vi "Save-modulation-data.vi"(8 "error in (no error)":errorcluster, 9 "Modulation data":i32[][](array[numeric]), 10 "File path":path) -> (0 "error out":errorcluster)   [LabVIEW 2013, in "MaterialCharacterization.lvlib" / "MC-SM1000.lvclass"]
uses:
  MC-SM1000.lvclass
  <vilib>/Utility/file.llb/Write To Spreadsheet File (I64).vi
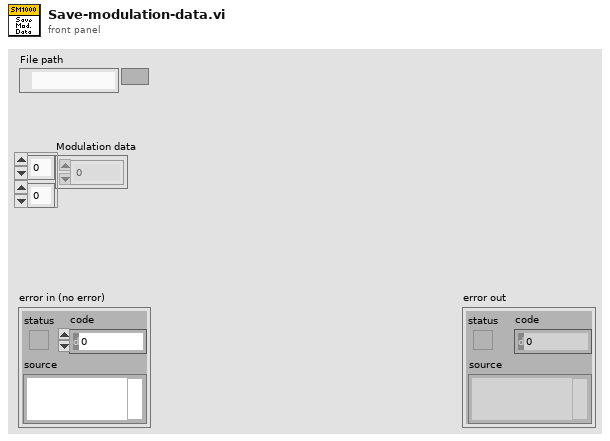
[diagram p1: front panel]
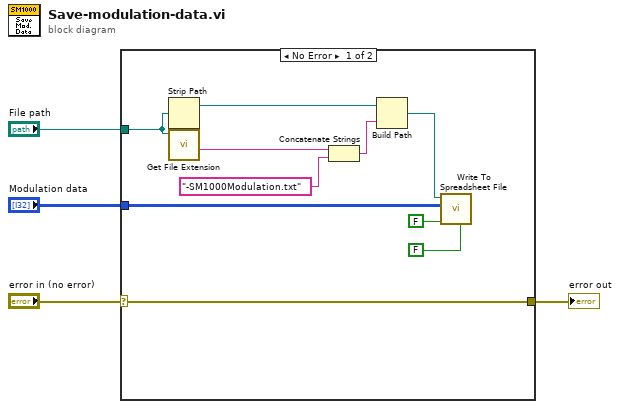
[diagram p0: block diagram]
diagram:
  n1 = case shown="No Error" "error in (no error)" {
    selector: "error in (no error)" -> [w8 w15]
    tunnel: [w8 w15] -> w3
    tunnel: "File path" -> [w7 _]
    tunnel: "Modulation data" -> [w14 _]
    frame No Error {
      n2 = Strip Path(path=w7) -> (stripped path=w12:path)  [unwired: 1 out]
      n3 = call <vilib>:"Get File Extension.vi"("file"=w7) -> ("filename without extension"=w5:string)  [unwired: 7 in, 3 out]
      n4 = Concatenate Strings(w5, "-SM1000Modulation.txt" ("string")) -> (w11:string)
      n5 = Build Path(base path=w12, name or relative path=w11) -> (appended path=w10:path)
      n6 = call-poly <vilib>:"Write To Spreadsheet File.vi"("transpose? (no:F)"=FALSE, "append to file? (new file:F)"=FALSE, "2D data"=w14, "file path (dialog if empty)"=w10) -> ()  [unwired: 4 in, 1 out]
    }
    frame Error {
    }
  }
  "error out" <- w3
